vi "TDT-Write Target (DBL).vi"(0 "Data":T1={"TTankX"=refnum, "TDevAccX"=refnum, "LastTime"=0.0, "error"={"status"=FALSE, "code"=0, "source"=""}, "Block Name"="", "Circuit Tag"="", "Tank Name"="", "NumTicks"=0, "LastTick"=0.0, "Idle?"=FALSE, "Wait (ms)"=1000, "LastArtf"=0.0, "LastTosc"=0.0}, 7 "Target":string, 9 "Val":dbl[](array[numeric]), 11 "error in (no error)":errorcluster) -> (15 "error out":errorcluster)   [LabVIEW 2015]
uses:
  TDT Interface Data.ctl
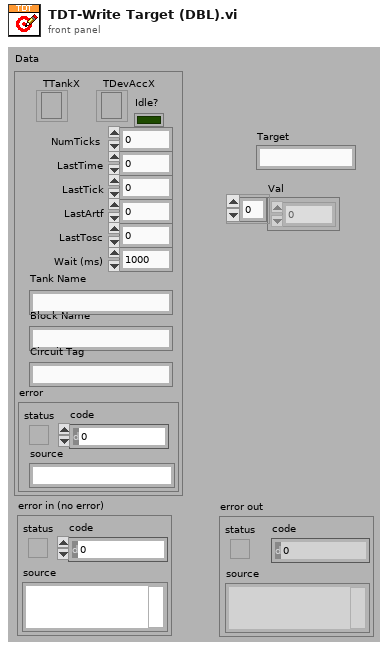
[diagram p1: front panel]
types:
  T1 = typedef "TDT Interface Data.ctl" = cluster{"TTankX":refnum<k7>, "TDevAccX":refnum<k7>, "LastTime":dbl, "error":errorcluster, "Block Name":string, "Circuit Tag":string, "Tank Name":string, "NumTicks":i32, "LastTick":dbl, "Idle?":bool, "Wait (ms)":u32, "LastArtf":dbl, "LastTosc":dbl}
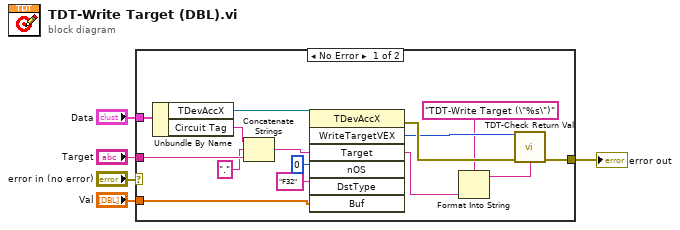
[diagram p0: block diagram]
diagram:
  n1 = case shown="No Error" "error in (no error)" {
    selector: "error in (no error)" -> [_ w21]
    tunnel: [w13 w21] -> w4
    tunnel: "Data" -> [w19 _]
    tunnel: "Target" -> [w17 _]
    tunnel: "Val" -> [w9 _]
    frame No Error {
      n2 = Unbundle By Name(w19) -> ("TDevAccX"=w20:refnum<k7>, "Circuit Tag"=w18:string)
      n3 = Concatenate Strings(w18, "." ("string"), w17) -> (w15:string)
      n4 = invoke class="TDevAccX" method="WriteTargetVEX"(reference=w20, "Target"=w15, "nOS"=0, "DstType"="F32", "Buf"=w9) -> (error out=w14:errorcluster, "WriteTargetVEX"=w12:i32, "Target"=w7:string)  [unwired: 2 in, 4 out]
      n5 = Format Into String(format string="TDT-Write Target (\"%s\")" ("source"), w7) -> (resulting string=w6:string)  [unwired: 2 in, 1 out]
      n6 = call "TDT-Check Return Val.vi"("Return Val"=w12, "error in (no error)"=w14, "source"=w6) -> ("error out"=w13:errorcluster)  [unwired: 12 in]
    }
    frame Error {
    }
  }
  "error out" <- w4
